vi "setUp.vi"(8 "error in (no error)":errorcluster, 11 "reference in":refnum<class "testcase-miscellaneous.lvclass">) -> (0 "error out":errorcluster, 3 "reference out":refnum<class "testcase-miscellaneous.lvclass">)   [LabVIEW 2017, in "testcase-miscellaneous.lvclass"]
doc: "setUp runs prior to the test method during test execution. Use this method to initialize any object data required by your tests."
uses:
  testcase-miscellaneous.lvclass
  C:/Program Files (x86)/National Instruments/LabVIEW 2017/vi.lib/addons/_JKI Toolkits/VI Tester/TestCase.llb/TestCase.lvclass
  testcase-miscellaneous.lvclass/testcase-miscellaneous.ctl
  <vilib>/addons/_JKI Toolkits/VI Tester/TestCase.llb/TestCase.lvclass
  src/examples/NEVSTOP/Communicable State Machine(CSM)/1. Create a reuse Module/1. Create a reuse Module.lvlib
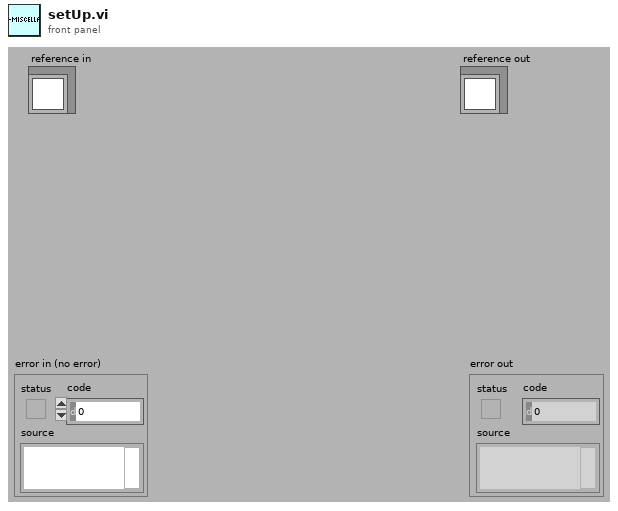
[diagram p1: front panel]
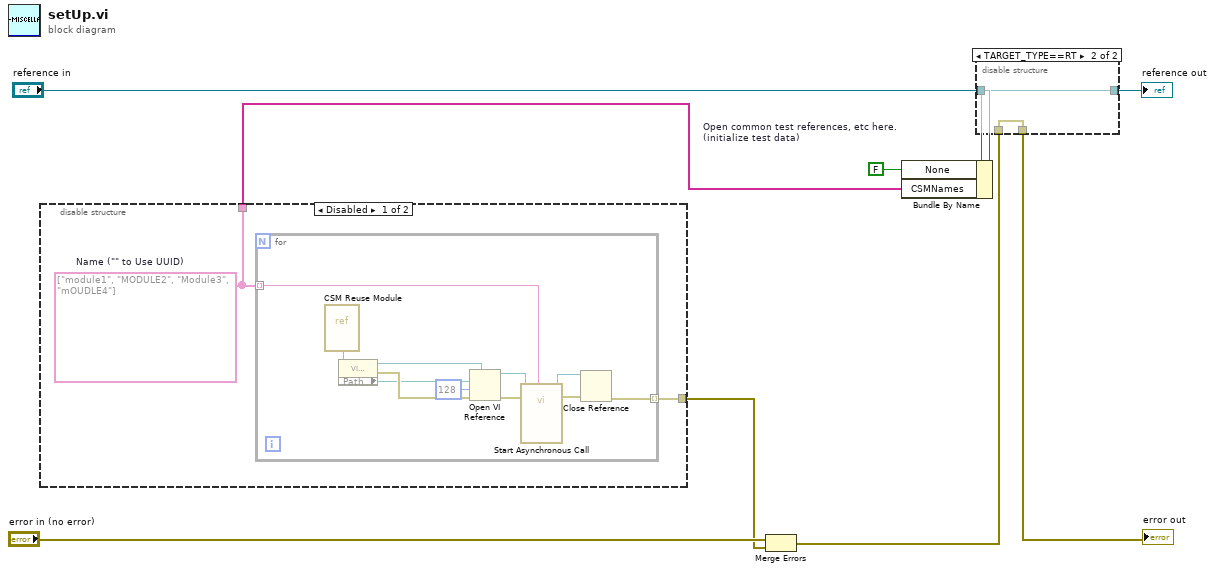
[diagram p0: block diagram]
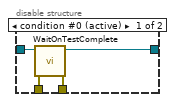
[diagram p3: hidden frame]
diagram:
  w4 = FALSE  # Open common test references, etc here. (initialize test data)
  n1 = disable-structure shown="Disabled" {
    disable-tunnel: [w11 _] -> w2
    disable-tunnel: [w10 _] -> w1
    frame Disabled {
      w10 = string[] ["module1", "MODULE2", "Module3", "mOUDLE4"]  # Name ("" to Use UUID)
      n2 = for {
        tunnel: w10 -> [w19] mode=indexing
        tunnel: [w12] -> w11 mode=indexing
        n3 = vi-ref "CSM Reuse Module.vi"() -> (w14:refnum<vi>)
        n4 = property class="VI (strict)"(reference=w14) -> (reference out=w18:refnum<vi>, error out=w16:errorcluster, "Path"=w15:path)  [unwired: 1 in]
        n5 = Open VI Reference(type specifier VI Refnum (for type only)=w18, vi path=w15, options=128, error in (no error)=w16) -> (vi reference=w17:refnum<vi>, error out=w13:errorcluster)  [unwired: 2 in]
        n6 = call-by-ref "Start Asynchronous Call"(reference=w17, error in=w13, "Name(\"\" to use uuid)"=w19) -> (reference out=w21:refnum<vi>, error out=w20:errorcluster)  [unwired: 11 in]
        n7 = Close Reference(reference=w21, error in (no error)=w20) -> (error out=w12:errorcluster)
      }
    }
    frame Enabled {
    }
  }
  n8 = Merge Errors("error in (no error)", w2) -> (w3:errorcluster)
  n9 = Bundle By Name(cluster="reference in", "None"=w4, "CSMNames"=w1) -> (w5:refnum<class "testcase-miscellaneous.lvclass">)
  n10 = disable-structure shown="TARGET_TYPE==RT" {
    disable-tunnel: w3 -> [w26 w27]
    disable-tunnel: [w25 w27] -> w8
    disable-tunnel: [w24 w28] -> w6
    disable-tunnel: w5 -> [w23 w28]
    frame condition #0 (active) {
      n11 = call <vilib>:"WaitOnTestComplete.vi"("error in (no error)"=w26, "TestCase in"=w23) -> ("error out"=w25:errorcluster, "TestCase out"=w24:refnum<class "testcase-miscellaneous.lvclass">)  [unwired: 8 in]
    }
    frame condition #1 {
    }
  }
  "error out" <- w8
  "reference out" <- w6
